vi "ep_Digital Data to U16 (N Samples).vi"(8 "error in":errorcluster, 11 "digital signal":bool[][](array[boolean])) -> (0 "error out":errorcluster, 3 "U16 digital data":u16[][](array[numeric])=[[0, 2], [0, 17]])   [LabVIEW 2011, in "NI_EP_COMTRADE.lvlib"]
uses:
  <vilib>/addons/Electrical Power/File IO/NI_EP_COMTRADE.lvlib
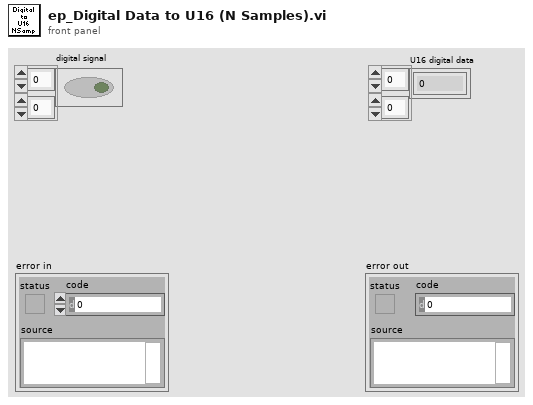
[diagram p1: front panel]
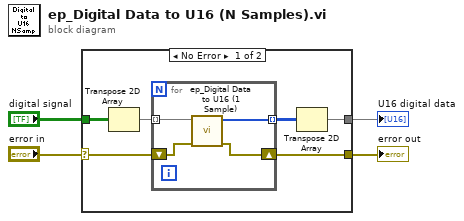
[diagram p0: block diagram]
diagram:
  n1 = case shown="No Error" "error in" {
    selector: "error in" -> [w6 w15]
    tunnel: "digital signal" -> [w10 _]
    tunnel: [w5 w15] -> w2
    tunnel: [w7 _] -> w1
    frame No Error {
      n2 = Transpose 2D Array(2D array=w10) -> (transposed array=w9:bool[][])
      n3 = for {
        tunnel: w9 -> [w14] mode=indexing
        tunnel: [w13] -> w8 mode=indexing
        shift-right: [w11] -> w5
        shift-left: w6 -> [w12]
        n4 = call <vilib>:"ep_Digital Data to U16 (1 Sample).vi"("error in"=w12, "digital signal"=w14) -> ("error out"=w11:errorcluster, "U16 digital data"=w13:u16[])  [unwired: 8 in]
      }
      n5 = Transpose 2D Array(2D array=w8) -> (transposed array=w7:u16[][])
    }
    frame Error {
    }
  }
  "error out" <- w2
  "U16 digital data" <- w1
